vi "Normalized Gaussian.vi"(8 "error in (no error)":errorcluster, 9 "width (c)":dbl, 10 "position (b)":dbl, 11 "Scale":dbl[](array[numeric])) -> (0 "error out":errorcluster, 3 "Normalized Gaussian":dbl[](array[numeric]))   [LabVIEW 2019, in "graph_utilities.lvclass"]
doc: "Normalized Gaussian."
uses:
  graph_utilities.lvclass
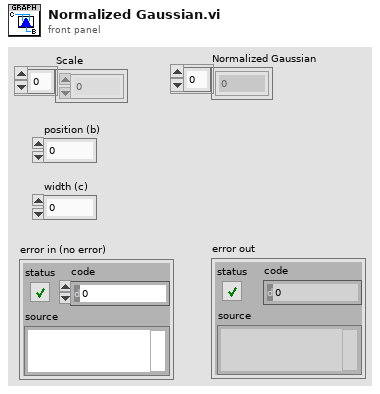
[diagram p1: front panel]
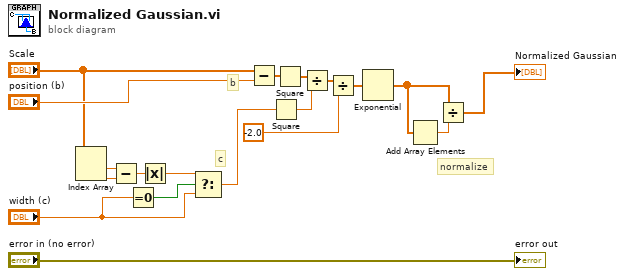
[diagram p0: block diagram]
diagram:
  # "c"
  # "normalize"
  # "b"
  n1 = Index Array(array="Scale") -> (element #1=w7:dbl, element #2=w6:dbl)  [unwired: 2 in]
  n2 = Subtract(x=w7, y=w6) -> (x-y=w5:dbl)
  n3 = Equal To 0?(x="width (c)") -> (x = 0?=w4:bool)
  n4 = Absolute Value(x=w5) -> (abs(x)=w3:dbl)
  n5 = Select(t=w3, s=w4, f="width (c)") -> (s? t:f=w1:dbl)
  n6 = Subtract(x="Scale", y="position (b)") -> (x-y=w12:dbl[])
  n7 = Square(x=w1) -> (x^2=w14:dbl)
  n8 = Square(x=w12) -> (x^2=w13:dbl[])
  n9 = Divide(x=w13, y=w14) -> (x/y=w15:dbl[])
  n10 = Divide(x=w15, y=-2.0 ("value")) -> (x/y=w17:dbl[])
  n11 = Exponential(1:w17) -> (0:w19:dbl[])
  n12 = Add Array Elements(numeric array=w19) -> (sum=w18:dbl)
  n13 = Divide(x=w19, y=w18) -> (x/y=→"Normalized Gaussian":dbl[])
  "error out" <- "error in (no error)"
